vi "Initialize.vi"(8 "error in":errorcluster, 10 "parameters":variant, 11 "Switch Channel in":refnum<class "Switch Channel.lvclass">) -> (0 "error out":errorcluster, 2 "summary":T2[](array[typedef]), 3 "data value reference":T1)   [LabVIEW 2025, in "Switch.lvlib" / "Switch Channel.lvclass"]
doc: "This Vi initializes the data of a node its default state.\nThe object is not created inside of this ViI, beacuase it is created from a File depending on user selection.Copyright 2017 National Instruments Corporation\n\nLicensed under the Apache License, Version 2.0 (the \"License\"); you may not use this file except in compliance with the License. You may obtain a copy of the License at http://www.apache.org/licenses/LICENSE-2.0\nUnless required by applicable law or agreed to in writing, software distributed under the License is distributed on an \"AS IS\" BASIS, WITHOUT WARRANTIES OR CONDITIONS OF ANY KIND, either express or implied. See the License for the specific language governing permissions and limitations under the License."
uses:
  Switch Channel.lvclass
  Users/Public/Documents/Sandia National Labs/TSS Plugin/CEF.lvlibp/Node/Summary.ctl
  Users/Public/Documents/Sandia National Labs/TSS Plugin/CEF.lvlibp/Node/NodeRef.ctl
  Users/Public/Documents/Sandia National Labs/TSS Plugin/CEF.lvlibp/Node/CEF_Node.lvclass
  Switch Channel.lvclass/Switch Channel.ctl
  Switch Channel configuration/Switch Channel configuration.lvclass
  C:/Users/Public/Documents/Sandia National Labs/TSS Plugin/Abstract Engine.lvlibp/Channel configuration/Channel configuration.lvclass
  Users/Public/Documents/Sandia National Labs/TSS Plugin/Abstract Engine.lvlibp/Channel configuration/Read Channel Setting.vi
  Users/Public/Documents/Sandia National Labs/TSS Plugin/Abstract Engine.lvlibp/Channel configuration/Write Channel Setting.vi
  Users/Public/Documents/Sandia National Labs/TSS Plugin/Abstract Engine.lvlibp/Abstract Channel/Abstract Channel.lvclass
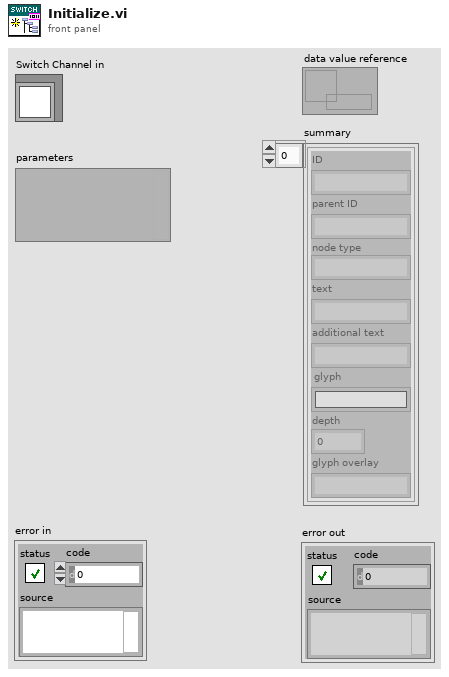
[diagram p1: front panel]
types:
  T1 = typedef "CEF.lvlibp/CEF_Node.lvclass/NodeRef.ctl" = refnum<data-value>
  T2 = typedef "CEF.lvlibp/CEF_Node.lvclass/Summary.ctl" = cluster{"ID":string, "parent ID":string, "node type":string, "text":string, "additional text":string, "glyph":string, "depth":i32, "glyph overlay":string}
  T3 = typedef "Abstract Engine.lvlibp/Channel configuration.lvclass/Default Channel.ctl" = cluster{"Address":string, "SW Alias":string, "Enabled":bool, "Type":string, "Description":string}
  T4 = cluster{"ID":string, "parent ID":string, "node type":string, "text":string, "additional text":string, "glyph":string, "depth":i32, "glyph overlay":string}[]
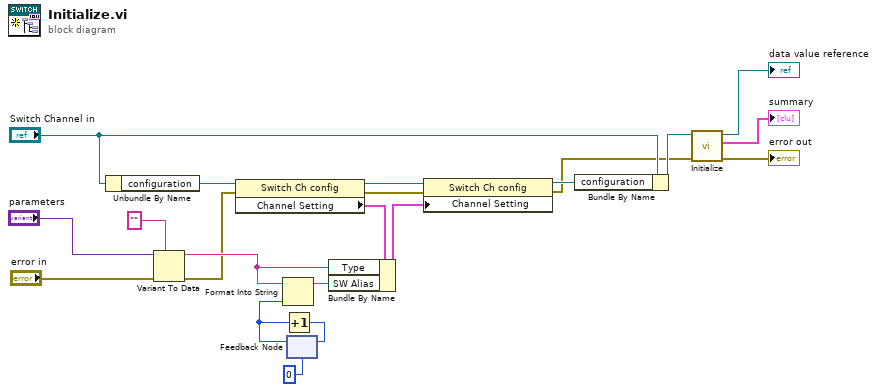
[diagram p0: block diagram]
diagram:
  n1 = Unbundle By Name("Switch Channel in") -> ("configuration"=w16:refnum<class "Switch Channel configuration.lvclass">)
  n2 = Variant To Data(error in="error in", type="" ("Class"), Variant="parameters") -> (data=w11:string, error out=w9:errorcluster)
  n3 = property class="Switch Ch config"(reference=w16, error in=w9) -> (reference out=w12:refnum<class "Switch Channel configuration.lvclass">, error out=w6:errorcluster, "Channel Setting"=w8:T3)
  n4 = feedback #1(0) -> (w4:i32)
  n5 = Format Into String(initial string=w11, w4) -> (resulting string=w2:string)  [unwired: 2 in, 1 out]
  n6 = Increment(x=w4) -> (x+1=w5:i32)
  n7 = feedback-in #1(w5) -> ()
  n8 = Bundle By Name(cluster=w8, "Type"=w11, "SW Alias"=w2) -> (w7:T3)
  n9 = property class="Switch Ch config"(reference=w12, error in=w6, "Channel Setting"=w7) -> (reference out=w14:refnum<class "Switch Channel configuration.lvclass">, error out=w10:errorcluster)
  n10 = Bundle By Name(cluster="Switch Channel in", "configuration"=w14) -> (w15:refnum<class "Switch Channel.lvclass">)
  n11 = call-parent "Initialize.vi"("error in"=w10, "CEF_Serialize node in"=w15) -> ("error out"=→"error out":errorcluster, "summary"=→"summary":T4, "data value reference"=→"data value reference":refnum<data-value>)  [unwired: 7 in]
